vi "CreateRespGate.vi"(8 "Gate Length":i32=250, 9 "Gate Start":i32=-150, 10 "Resp Marks":i32[][](array[numeric]), 11 "Lines":i32=250) -> (3 "Resp Gate":bool[][](array[boolean]))   [LabVIEW 2022 SP3]
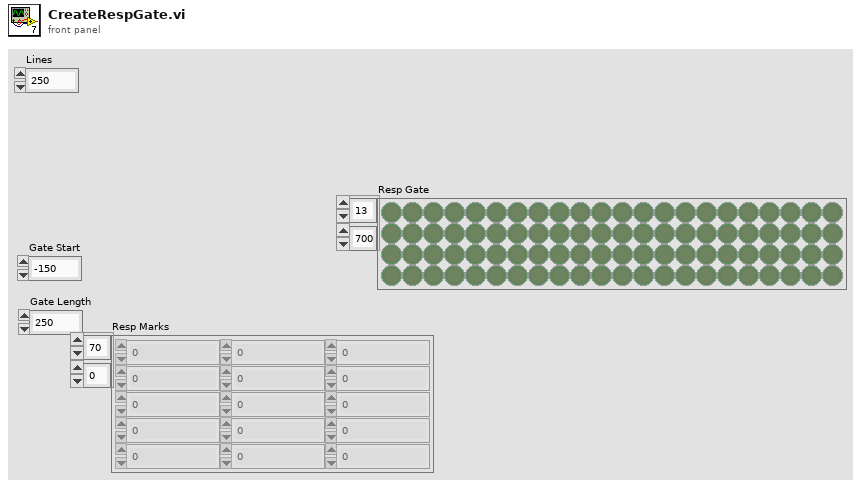
[diagram p1: front panel]
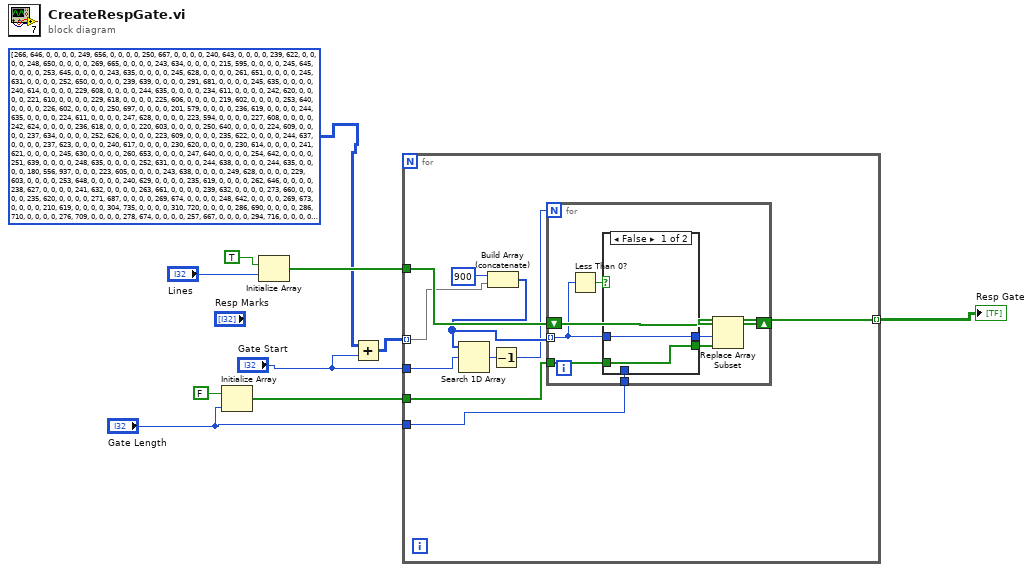
[diagram p0: block diagram]
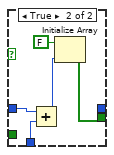
[diagram p2: hidden frame]
diagram:
  n1 = Initialize Array(FALSE, "Gate Length") -> (w4:bool[])
  n2 = Initialize Array(TRUE, "Lines") -> (w8:bool[])
  n3 = Add(x=i32[][] [[266, 646, 0, 0, 0, 0], [249, 656, 0, 0, 0, 0], [250, 667, 0, 0, 0, 0], [240, 643, 0, 0, 0, 0], [239, 622, 0, 0, 0, 0], [248, 650, 0, 0, 0, 0], [269, 665, 0, 0, 0, 0], [243, 634, 0, 0, 0, 0], [215, 595, 0, 0, 0, 0], [245, 645, 0, 0, 0, 0], [253, 645, 0, 0, 0, 0], [243, 635, 0, 0, 0, 0], [245, 628, 0, 0, 0, 0], [261, 651, 0, 0, 0, 0], [245, 631, 0, 0, 0, 0], [252, 650, 0, 0, 0, 0], [239, 639, 0, 0, 0, 0], [291, 681, 0, 0, 0, 0], [245, 635, 0, 0, 0, 0], [240, 614, 0, 0, 0, 0], [229, 608, 0, 0, 0, 0], [244, 635, 0, 0, 0, 0], [234, 611, 0, 0, 0, 0], [242, 620, 0, 0, 0, 0], [221, 610, 0, 0, 0, 0], [229, 618, 0, 0, 0, 0], [225, 606, 0, 0, 0, 0], [219, 602, 0, 0, 0, 0], [253, 640, 0, 0, 0, 0], [226, 602, 0, 0, 0, 0], [250, 697, 0, 0, 0, 0], [201, 579, 0, 0, 0, 0], [236, 619, 0, 0, 0, 0], [244, 635, 0, 0, 0, 0], [224, 611, 0, 0, 0, 0], [247, 628, 0, 0, 0, 0], [223, 594, 0, 0, 0, 0], [227, 608, 0, 0, 0, 0], [242, 624, 0, 0, 0, 0], [236, 618, 0, 0, 0, 0], [220, 603, 0, 0, 0, 0], [250, 640, 0, 0, 0, 0], [224, 609, 0, 0, 0, 0], [237, 634, 0, 0, 0, 0], [252, 626, 0, 0, 0, 0], [223, 609, 0, 0, 0, 0], [235, 622, 0, 0, 0, 0], [244, 637, 0, 0, 0, 0], [237, 623, 0, 0, 0, 0], [240, 617, 0, 0, 0, 0], [230, 620, 0, 0, 0, 0], [230, 614, 0, 0, 0, 0], [241, 621, 0, 0, 0, 0], [245, 630, 0, 0, 0, 0], [260, 653, 0, 0, 0, 0], [247, 640, 0, 0, 0, 0], [254, 642, 0, 0, 0, 0], [251, 639, 0, 0, 0, 0], [248, 635, 0, 0, 0, 0], [252, 631, 0, 0, 0, 0], [244, 638, 0, 0, 0, 0], [244, 635, 0, 0, 0, 0], [180, 556, 937, 0, 0, 0], [223, 605, 0, 0, 0, 0], [243, 638, 0, 0, 0, 0], [249, 628, 0, 0, 0, 0], [229, 603, 0, 0, 0, 0], [253, 648, 0, 0, 0, 0], [240, 629, 0, 0, 0, 0], [235, 619, 0, 0, 0, 0], [262, 646, 0, 0, 0, 0], [238, 627, 0, 0, 0, 0], [241, 632, 0, 0, 0, 0], [263, 661, 0, 0, 0, 0], [239, 632, 0, 0, 0, 0], [273, 660, 0, 0, 0, 0], [235, 620, 0, 0, 0, 0], [271, 687, 0, 0, 0, 0], [269, 674, 0, 0, 0, 0], [248, 642, 0, 0, 0, 0], [269, 673, 0, 0, 0, 0], [210, 619, 0, 0, 0, 0], [304, 735, 0, 0, 0, 0], [310, 720, 0, 0, 0, 0], [286, 690, 0, 0, 0, 0], [286, 710, 0, 0, 0, 0], [276, 709, 0, 0, 0, 0], [278, 674, 0, 0, 0, 0], [257, 667, 0, 0, 0, 0], [294, 716, 0, 0, 0, 0], [285, 715, 0, 0, 0, 0], [292, 717, 0, 0, 0, 0], [299, 726, 0, 0, 0, 0], [294, 726, 0, 0, 0, 0], [298, 699, 0, 0, 0, 0], [255, 657, 0, 0, 0, 0], [268, 664, 0, 0, 0, 0], [294, 707, 0, 0, 0, 0], [279, 712, 0, 0, 0, 0], [307, 737, 0, 0, 0, 0], [282, 708, 0, 0, 0, 0], [292, 702, 0, 0, 0, 0], [284, 726, 0, 0, 0, 0], [300, 738, 0, 0, 0, 0], [296, 724, 0, 0, 0, 0], [277, 692, 0, 0, 0, 0], [263, 688, 0, 0, 0, 0], [303, 740, 0, 0, 0, 0], [301, 717, 0, 0, 0, 0], [278, 711, 0, 0, 0, 0], [296, 725, 0, 0, 0, 0], [296, 723, 0, 0, 0, 0], [294, 728, 0, 0, 0, 0], [310, 762, 0, 0, 0, 0], [286, 695, 0, 0, 0, 0], [281, 705, 0, 0, 0, 0], [283, 717, 0, 0, 0, 0], [307, 746, 0, 0, 0, 0], [282, 712, 0, 0, 0, 0], [281, 698, 0, 0, 0, 0], [280, 722, 0, 0, 0, 0], [304, 761, 0, 0, 0, 0], [321, 767, 0, 0, 0, 0], [312, 743, 0, 0, 0, 0], [290, 726, 0, 0, 0, 0], [293, 726, 0, 0, 0, 0], [295, 710, 0, 0, 0, 0], [304, 756, 0, 0, 0, 0], [313, 755, 0, 0, 0, 0], [306, 758, 0, 0, 0, 0], [298, 732, 0, 0, 0, 0], [317, 762, 0, 0, 0, 0], [326, 774, 0, 0, 0, 0], [309, 733, 0, 0, 0, 0], [295, 737, 0, 0, 0, 0], [299, 745, 0, 0, 0, 0], [316, 774, 0, 0, 0, 0], [330, 798, 0, 0, 0, 0], [309, 750, 0, 0, 0, 0], [301, 738, 0, 0, 0, 0], [311, 761, 0, 0, 0, 0], [316, 767, 0, 0, 0, 0], [334, 799, 0, 0, 0, 0], [321, 789, 0, 0, 0, 0], [291, 736, 0, 0, 0, 0], [297, 744, 0, 0, 0, 0], [309, 732, 0, 0, 0, 0], [334, 795, 0, 0, 0, 0], [314, 786, 0, 0, 0, 0], [332, 806, 0, 0, 0, 0], [329, 788, 0, 0, 0, 0], [332, 763, 0, 0, 0, 0], [300, 765, 0, 0, 0, 0], [347, 804, 0, 0, 0, 0], [332, 803, 0, 0, 0, 0], [326, 791, 0, 0, 0, 0], [316, 768, 0, 0, 0, 0], [323, 775, 0, 0, 0, 0], [346, 821, 0, 0, 0, 0], [345, 811, 0, 0, 0, 0], [338, 785, 0, 0, 0, 0]] ("Resp"), y="Gate Start") -> (x+y=w3:i32[][])
  n4 = for {
    tunnel: "Gate Length" -> [w20]
    tunnel: [w19] -> w10 mode=indexing
    tunnel: w8 -> [w18]
    tunnel: w4 -> [w17]
    tunnel: w3 -> [w14] mode=indexing
    tunnel: "Gate Start" -> [w12]
    n5 = Build Array (concatenate)(900, w14) -> (w13:i32[])
    n6 = Search 1D Array(1D array=w13, element=w12) -> (index of element=w16:i32)  [unwired: 1 in]
    n7 = Decrement(x=w16) -> (x-1=w11:i32)
    n8 = for {
      N: w11 -> [_]
      tunnel: w13 -> [w23] mode=indexing
      shift-right: [w27] -> w19
      shift-left: w18 -> [w28]
      tunnel: w17 -> [w24]
      tunnel: w20 -> [w22]
      n9 = Less Than 0?(x=w23) -> (x < 0?=w26:bool)
      n10 = case shown="False" w26 {
        tunnel: [w30 w31] -> w25
        tunnel: w24 -> [w30 _]
        tunnel: w23 -> [w29 w35]
        tunnel: w22 -> [_ w34]
        tunnel: [w29 _] -> w21
        frame False {
        }
        frame True {
          n11 = Add(x=w35, y=w34) -> (x+y=w32:i32)
          n12 = Initialize Array(FALSE, w32) -> (w31:bool[])
        }
      }
      n13 = Replace Array Subset(array=w28, new element=w25, index=w21) -> (w27:bool[])
    }
  }
  "Resp Gate" <- w10
